vi "Error Read.vi"(8 "error in":errorcluster, 11 "Power Supply In":refnum<class "Power Supply.lvclass">) -> (0 "error out":errorcluster, 1 "Changed or First Call?":bool, 2 "Error Acknowledge ACT":bool, 3 "Power Supply Out":refnum<class "Power Supply.lvclass">)   [LabVIEW 2023, in "Power Supply.lvclass"]
uses:
  Power Supply.lvclass
  Power Supply.lvclass/Power Supply.ctl
  Low Level Capabilities/Error/Error.lvclass
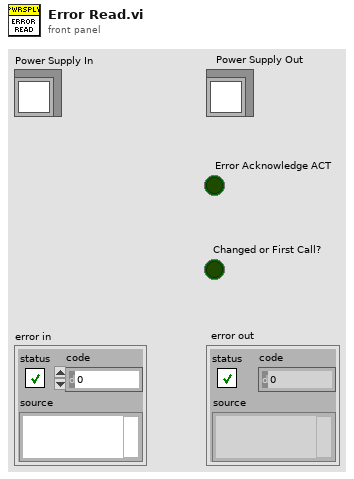
[diagram p1: front panel]
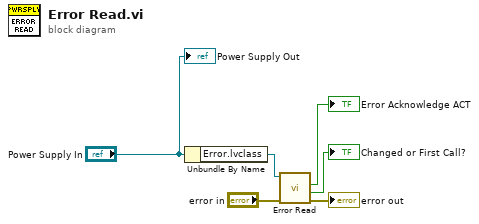
[diagram p0: block diagram]
diagram:
  n1 = Unbundle By Name("Power Supply In") -> ("Error.lvclass"=w5:refnum<class "Error.lvclass">)
  n2 = call-dynamic "Error Read.vi"("error in"="error in", "Error in"=w5) -> ("error out"=→"error out":errorcluster, "Changed or First Call?"=→"Changed or First Call?":bool, "Error Acknowledge ACT"=→"Error Acknowledge ACT":bool)  [unwired: 6 in, 1 out]
  "Power Supply Out" <- "Power Supply In"
